vi "Display Hardware Devices.vi"(8 "error in (no error)":errorcluster, 9 "Hardware Type":string, 10 "Array of Hardware Device Names":string[](array[string]), 11 "Operator UI in":refnum<class "Measurement UI.lvclass">) -> (0 "error out":errorcluster, 3 "Operator UI out":refnum<class "Measurement UI.lvclass">)   [LabVIEW 2015, in "Measurement UI.lvlib" / "Measurement UI.lvclass"]
uses:
  Measurement UI.lvclass
  Measurement UI.lvclass/Measurement UI.ctl
  Accessors/Read Digitizer.vi
  Accessors/Read Function Generator.vi
  Accessors/Read Power Supply.vi
  Read Multimeter.vi
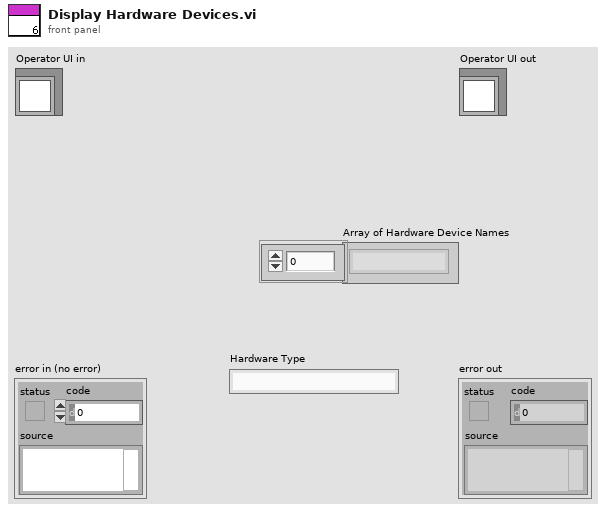
[diagram p1: front panel]
types:
  T1 = enum8{"Enabled", "Disabled", "Disabled and Grayed Out"}
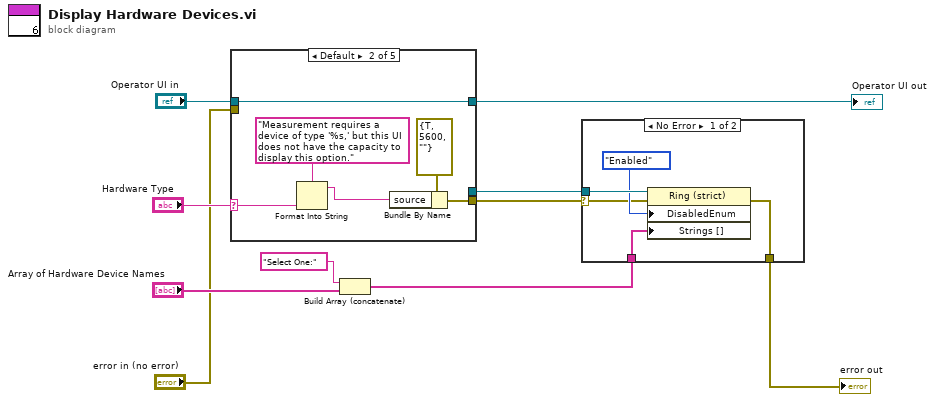
[diagram p0: block diagram]
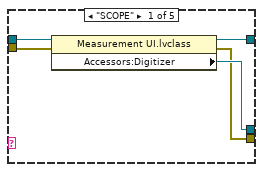
[diagram p3: hidden frame]
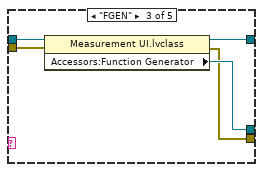
[diagram p4: hidden frame]
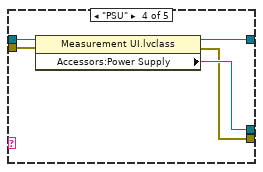
[diagram p5: hidden frame]
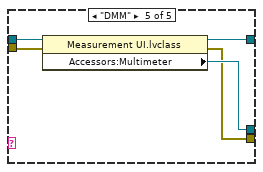
[diagram p6: hidden frame]
diagram:
  n1 = case shown="Default" "Hardware Type" {
    selector: "Hardware Type" -> [_ w18 _ _ _]
    tunnel: [w13 _ w24 w29 w36] -> w6
    tunnel: "Operator UI in" -> [w15 w21 w26 w31 w35]
    tunnel: [w14 w21 w25 w30 w34] -> w3
    tunnel: "error in (no error)" -> [w11 _ w23 w28 w32]
    tunnel: [w12 w19 w22 w27 w33] -> w1
    frame "SCOPE" {
      n2 = property class="Measurement UI.lvclass"(reference=w15, error in=w11) -> (reference out=w14:refnum<class "Measurement UI.lvclass">, error out=w12:errorcluster, "Accessors:Digitizer"=w13:refnum<vi>)
    }
    frame Default {
      n3 = Format Into String(format string="Measurement requires a device of type '%s,' but this UI does not have the capacity to display this option.", w18) -> (resulting string=w17:string)  [unwired: 2 in, 1 out]
      n4 = Bundle By Name(cluster=errorcluster {"status"=TRUE, "code"=5600, "source"=""} ("error out"), "source"=w17) -> (w19:errorcluster)
    }
    frame "FGEN" {
      n5 = property class="Measurement UI.lvclass"(reference=w26, error in=w23) -> (reference out=w25:refnum<class "Measurement UI.lvclass">, error out=w22:errorcluster, "Accessors:Function Generator"=w24:refnum<vi>)
    }
    frame "PSU" {
      n6 = property class="Measurement UI.lvclass"(reference=w31, error in=w28) -> (reference out=w30:refnum<class "Measurement UI.lvclass">, error out=w27:errorcluster, "Accessors:Power Supply"=w29:refnum<vi>)
    }
    frame "DMM" {
      n7 = property class="Measurement UI.lvclass"(reference=w35, error in=w32) -> (reference out=w34:refnum<class "Measurement UI.lvclass">, error out=w33:errorcluster, "Accessors:Multimeter"=w36:refnum<vi>)
    }
  }
  "Operator UI out" <- w3
  n8 = Build Array (concatenate)("Select One:" ("String"), "Array of Hardware Device Names") -> (w7:string[])
  n9 = case shown="No Error" w1 {
    selector: w1 -> [w37 w42]
    tunnel: w7 -> [w41 _]
    tunnel: w6 -> [w40 _]
    tunnel: [w38 w42] -> w4
    frame No Error {
      n10 = property class="Ring (strict)"(reference=w40, error in=w37, "DisabledEnum"=T1."Enabled" ("Disabled"), "Strings []"=w41) -> (error out=w38:errorcluster)  [unwired: 1 out]
    }
    frame Error {
    }
  }
  "error out" <- w4
